vi "Flatten.vi"(8 "error in (no error)":errorcluster, 11 "Translation Stage in":refnum<class "Translation Stage.lvclass">) -> (0 "error out":errorcluster, 3 "Translation Stage out":refnum<class "Translation Stage.lvclass">)   [LabVIEW 2023, in "Translation Stage.lvclass"]
uses:
  Translation Stage.lvclass
  Translation Stage.lvclass/Translation Stage.ctl
  Global/File Locations.vi
  Scanner/Scanner.lvclass
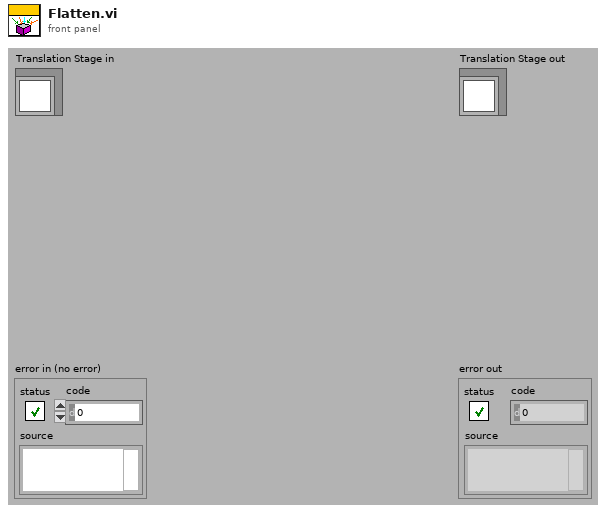
[diagram p1: front panel]
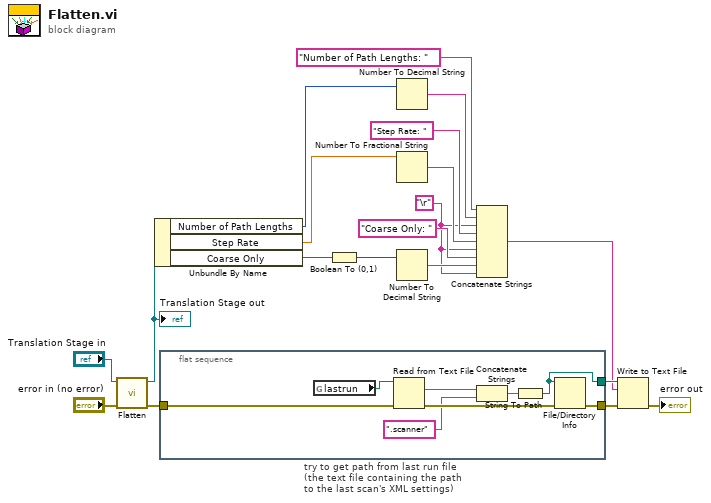
[diagram p0: block diagram]
diagram:
  w2 = "\r"
  n1 = call-parent "Flatten.vi"("error in (no error)"="error in (no error)", "Scanner in"="Translation Stage in") -> ("error out"=w17:errorcluster, "Scanner out"=w13:refnum<class "Translation Stage.lvclass">)  [unwired: 8 in]
  "Translation Stage out" <- w13
  n2 = Unbundle By Name(w13) -> ("Number of Path Lengths"=w11:i32, "Step Rate"=w12:dbl, "Coarse Only"=w9:bool)
  n3 = flat-sequence "try to get path from last run file\n(the text file containing the path\nto the last scan's XML settings)" {
    tunnel: [w27] -> w14
    tunnel: [w24] -> w15
    tunnel: w17 -> [w23]
    frame #0 {
      n4 = global read "File Locations.vi" "lastrun"() -> (w26:path)
      n5 = Read from Text File(file (use dialog)=w26, error in=w23) -> (text=w22:string, error out=w25:errorcluster)  [unwired: 4 out]
      n6 = Concatenate Strings(w22, ".scanner") -> (w20:string)
      n7 = String To Path(string=w20) -> (path=w27:path)
      n8 = File/Directory Info(path=w27, error in=w25) -> (error out=w24:errorcluster)  [unwired: 6 out]
    }
  }
  n9 = Boolean To (0,1)(Boolean=w9) -> (0, 1=w10:i16)
  n10 = Number To Decimal String(number=w11) -> (decimal integer string=w7:string)  [unwired: 1 in]
  n11 = Number To Fractional String(number=w12) -> (F-format string=w5:string)  [unwired: 3 in]
  n12 = Number To Decimal String(number=w10) -> (decimal integer string=w3:string)  [unwired: 1 in]
  n13 = Concatenate Strings("Number of Path Lengths: ", w7, w2, "Step Rate: ", w5, w2, "Coarse Only: ", w3, w2) -> (w1:string)
  n14 = Write to Text File(file (use dialog)=w14, text=w1, error in=w15) -> (error out=→"error out":errorcluster)  [unwired: 1 in, 2 out]
